vi "RWText.vi"(7 "Action":enum16{"Read", "Write"}(ring), 8 "error in":errorcluster, 10 "TextIn":string, 11 "file path (use dialog)":path) -> (0 "error out":errorcluster, 2 "textOut":string)   [LabVIEW 2019]
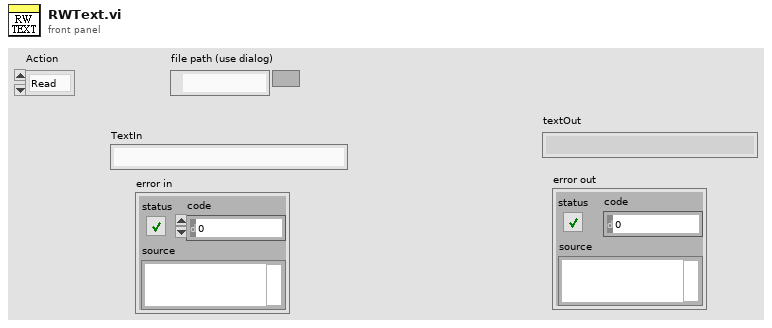
[diagram p1: front panel]
types:
  T1 = enum16{"open", "replace", "create", "open or create", "replace or create", "replace or create with confirmation"}
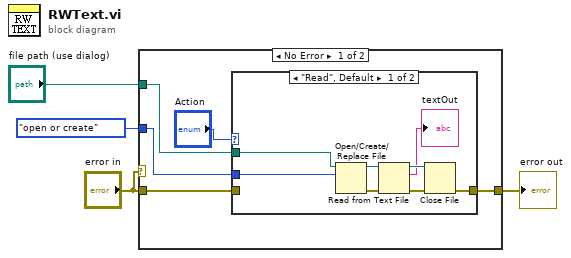
[diagram p0: block diagram]
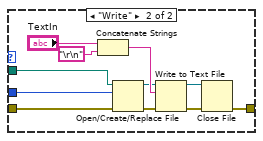
[diagram p2: hidden frame]
diagram:
  n1 = case shown="No Error" "error in" {
    tunnel: "error in" -> [w9 w29]
    tunnel: [w8 w29] -> w3
    tunnel: "file path (use dialog)" -> [w7 _]
    tunnel: T1."open or create" ("operation (0:open)") -> [w5 _]
    frame No Error {
      n2 = case shown="\"Read\", Default" "Action" {
        tunnel: w9 -> [_ w21]
        tunnel: [w11 w20] -> w8
        tunnel: w7 -> [w17 w19]
        tunnel: w5 -> [w16 w18]
        frame "Read", Default {
          n3 = Open/Create/Replace File(file path (use dialog)=w17, operation (0:open)=w16) -> (refnum out=w15:refnum<file>, error out=w14:errorcluster)  [unwired: 4 in, 1 out]
          n4 = Read from Text File(file (use dialog)=w15, error in=w14) -> (refnum out=w13:refnum<file>, text=→"textOut":string, error out=w12:errorcluster)  [unwired: 2 in, 1 out]
          n5 = Close File(refnum=w13, error in=w12) -> (error out=w11:errorcluster)  [unwired: 1 out]
        }
        frame "Write" {
          n6 = Concatenate Strings("TextIn", "\r\n") -> (w26:string)
          n7 = Open/Create/Replace File(file path (use dialog)=w19, error in=w21, operation (0:open)=w18) -> (refnum out=w22:refnum<file>, error out=w23:errorcluster)  [unwired: 3 in, 1 out]
          n8 = Write to Text File(file (use dialog)=w22, text=w26, error in=w23) -> (refnum out=w28:refnum<file>, error out=w27:errorcluster)  [unwired: 1 in, 1 out]
          n9 = Close File(refnum=w28, error in=w27) -> (error out=w20:errorcluster)  [unwired: 1 out]
        }
      }
    }
    frame Error {
    }
  }
  "error out" <- w3
